vi "BUSY.vi"(3 "error in":errorcluster, 4 "Stage Axis":string, 5 "Offset":dbl, 6 "VISA Stage":refnum<visa-resource-name>) -> (0 "error out":errorcluster, 1 "position":dbl, 2 "read buffer":string)   [LabVIEW 2011]
uses:
  GLOBAL.vi
panel:
  in  "Case Constant":bool=TRUE
  out "target":i32
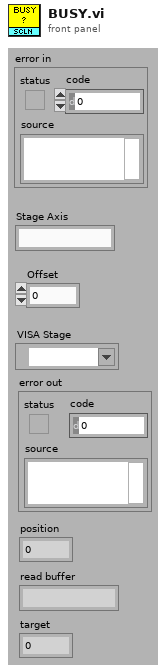
[diagram p1: front panel]
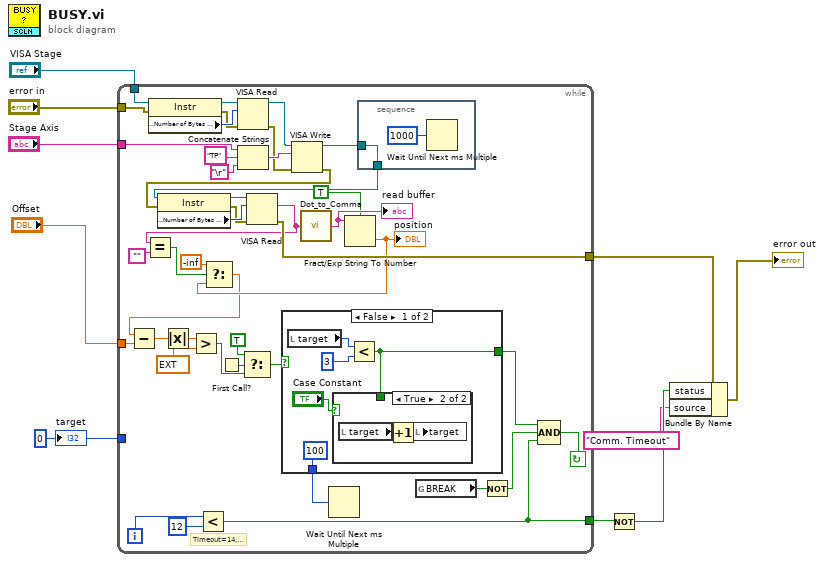
[diagram p0: block diagram]
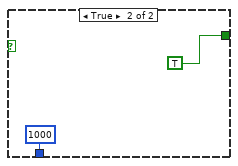
[diagram p3: hidden frame]
diagram:
  w6 = 0 ("target")
  n1 = while {
    tunnel: "VISA Stage" -> [w28]
    tunnel: "Offset" -> [w51]
    tunnel: "Stage Axis" -> [w52]
    tunnel: [w39] -> w5
    tunnel: "error in" -> [w27]
    tunnel: w6 -> [_]
    tunnel: [w12] -> w3
    i -> [w14]
    stop <- w15 continue-if-true
    # "Timeout=14,4s"
    n2 = property class="Instr"(reference=w28, error in=w27) -> (reference out=w29:refnum<visa-resource-name>, error out=w30:errorcluster, "Serial Settings:Number of Bytes at Serial Port"=w31:u32)
    n3 = Less?(x=w14, y=12) -> (x < y?=w12:bool)
    n4 = First Call?() -> (First Call?: T/F=w38:bool)
    n5 = VISA Read(VISA resource name=w29, byte count=w31, error in (no error)=w30) -> (VISA resource name out=w26:refnum<visa-resource-name>, error out=w25:errorcluster)  [unwired: 2 out]
    n6 = Concatenate Strings(w52, "TP" ("string"), "\r") -> (w50:string)
    n7 = VISA Write(VISA resource name=w26, write buffer=w50, error in (no error)=w25) -> (VISA resource name out=w34:refnum<visa-resource-name>, error out=w45:errorcluster)  [unwired: 1 out]
    n8 = stacked-sequence {
      tunnel: w34 -> [w53]
      tunnel: [w53] -> w33
      frame #0 {
        n9 = Wait Until Next ms Multiple(millisecond multiple=u32 1000 ("milliseconds to wait")) -> ()  [unwired: 1 out]
      }
    }
    n10 = property class="Instr"(reference=w33, error in=w45) -> (reference out=w46:refnum<visa-resource-name>, error out=w47:errorcluster, "Serial Settings:Number of Bytes at Serial Port"=w48:u32)
    n11 = VISA Read(VISA resource name=w46, byte count=w48, error in (no error)=w47) -> (read buffer=w23:string, error out=w39:errorcluster)  [unwired: 2 out]
    n12 = Equal?(x=w23, y="") -> (x = y?=w22:bool)
    n13 = call "Dot_to_Comma.vi"("String in"=w23) -> ("String out"=w40:string)
    "read buffer" <- w40
    n14 = Fract/Exp String To Number(use system decimal point (T)=TRUE, string=w40) -> (number=w21:dbl)  [unwired: 3 out]
    "position" <- w21
    n15 = Select(t=-inf, s=w22, f=w21) -> (s? t:f=w20:dbl)
    n16 = Subtract(x=w20, y=w51) -> (x-y=w44:dbl)
    n17 = Absolute Value(x=w44) -> (abs(x)=w43:dbl)
    n18 = Greater?(x=w43, y=ext 0.005) -> (0:w37:bool)
    n19 = Select(t=TRUE, s=w38, f=w37) -> (s? t:f=w35:bool)
    n20 = case shown="False" w35 {
      tunnel: [w56 TRUE] -> w16
      tunnel: [u32 100 ("y") u32 1000 ("y")] -> w32
      frame False {
        n21 = local read "target"() -> (w58:i32)
        n22 = Less?(x=w58, y=3) -> (x < y?=w56:bool)
        n23 = case shown="True" "Case Constant" {
          tunnel: w56 -> [_ _]
          frame False {
          }
          frame True {
            n24 = local read "target"() -> (w61:i32)
            n25 = Increment(x=w61) -> (x+1=w60:i32)
            n26 = local write "target"(w60) -> ()
          }
        }
      }
      frame True {
      }
    }
    n27 = Wait Until Next ms Multiple(millisecond multiple=w32) -> ()  [unwired: 1 out]
    n28 = global read "GLOBAL.vi" "BREAK"() -> (w18:bool)
    n29 = Not(x=w18) -> (.not. x?=w17:bool)
    n30 = Compound Arithmetic op=AND(w16, w17, w12) -> (w15:bool)
  }
  n31 = Not(x=w3) -> (.not. x?=w2:bool)
  n32 = Bundle By Name(cluster=w5, "status"=w2, "source"="Comm. Timeout") -> (→"error out":errorcluster)
  "target" <- w6
